vi "Color Space Test.vi"() -> ()   [LabVIEW 2013]
panel:
  out "2D Picture":picture
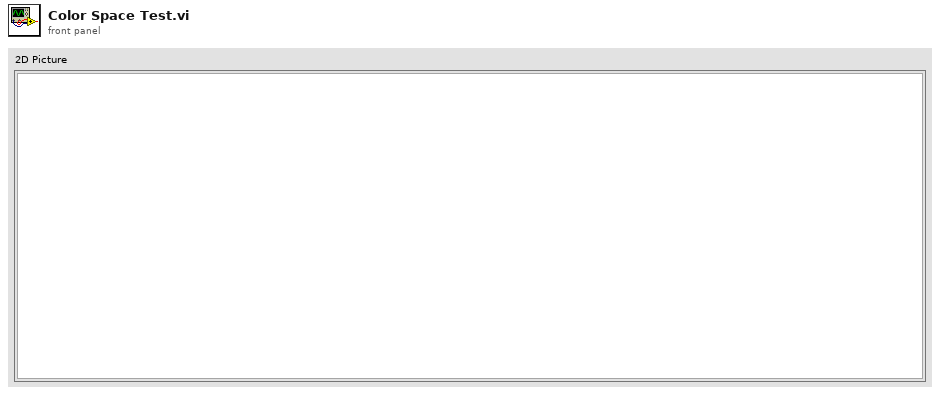
[diagram p1: front panel]
types:
  T1 = cluster{"left":i16, "top":i16, "right":i16, "bottom":i16}
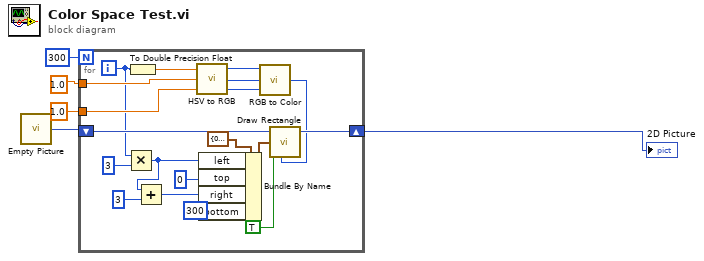
[diagram p0: block diagram]
diagram:
  n1 = call "Empty Picture"() -> ("empty picture"=w2:picture)
  n2 = for {
    N: 300 -> [_]
    tunnel: 1.0 -> [w24]
    tunnel: 1.0 -> [w23]
    shift-right: [w21] -> w1
    shift-left: w2 -> [w22]
    i -> [w7]
    n3 = Multiply(x=w7, y=3) -> (x*y=w18:i32)
    n4 = To Double Precision Float(number=w7) -> (double precision float=w6:dbl)
    n5 = Add(x=w18, y=3) -> (x+y=w16:i32)
    n6 = call "HSV to RGB.vi"("V"=w23, "S"=w24, "H"=w6) -> ("B"=w10:u8, "G"=w11:u8, "R"=w12:u8)
    n7 = Bundle By Name(cluster=T1 {"left"=0, "top"=0, "right"=0, "bottom"=0} ("rect"), "left"=w18, "top"=i16 0, "right"=w16, "bottom"=i16 300) -> (w13:T1)
    n8 = call <vilib>:"RGB to Color.vi"("B"=w10, "G"=w11, "R"=w12) -> ("Color"=w9:u32)
    n9 = call <vilib>:"Draw Rectangle.vi"("picture"=w22, "rect"=w13, "fill?(F)"=TRUE, "color(black)"=w9) -> ("new picture"=w21:picture)  [unwired: 5 in]
  }
  "2D Picture" <- w1
